vi "PIV_transform.vi"(8 "error in (no error)":errorcluster, 11 "raw":T1) -> (0 "error out":errorcluster={"status"=TRUE, "code"=1671, "source"="Python Node in PIV_Pixel.vi->LabVIEW_GUI.vi<APPEND>\n\nModule Path: /Users/crogers/Desktop/PIV/LabVIEW/subs/code.py\nFunction Name: piv\nPython returned the following error: <class 'OSError'>\nImageIO does not generally support reading folders. Limited support may be available via specific plugins. Specify the plugin explicitly using the `plugin` kwarg, e.g. `plugin='DICOM'`\n\n\n Call Stack information:\n['Traceback (most recent call last):\n', '  File \"/Users/crogers/Desktop/PIV/LabVIEW/subs/code.py\", line 8, in piv\n    frame_a = tools.imread(path_t)\n', '  File \"/Users/crogers/Library/Python/3.10/lib/python/site-packages/openpiv/tools.py\", line 337, in imread\n    im = _imread(filename)\n', '  File \"/Users/crogers/Library/Python/3.10/lib/python/site-packages/imageio/v3.py\", line 53, in imread\n    with imopen(uri, \"r\", **plugin_kwargs) as img_file:\n', '  File \"/Users/crogers/Library/Python/3.10/lib/python/site-packages/imageio/core/imopen.py\", line 223, in imopen\n    raise err_type(err_msg)\n', \"OSError: ImageIO does not generally support reading folders. Limited support may be available via specific plugins. Specify the plugin explicitly using the `plugin` kwarg, e.g. `plugin='DICOM'`\n\"]"}, 3 "interpolated":T1)   [LabVIEW 2025]
uses:
  PIV_velocities.ctl
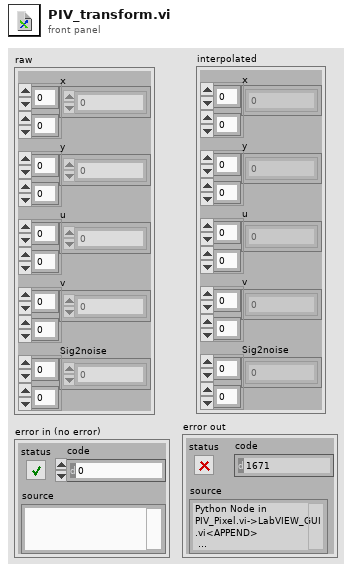
[diagram p1: front panel]
types:
  T1 = typedef "PIV_velocities.ctl" = cluster{"x":dbl[][], "y":dbl[][], "u":dbl[][], "v":dbl[][], "Sig2noise":dbl[][]}
  T2 = cluster{"x":dbl[][], "y":dbl[][], "u3":dbl[][], "v3":dbl[][]}
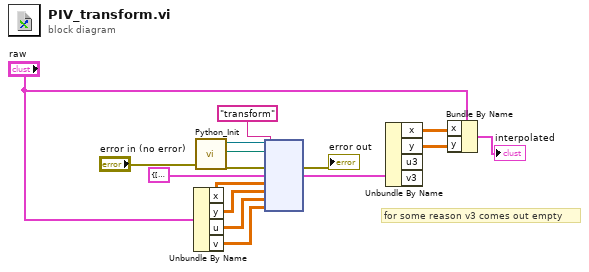
[diagram p0: block diagram]
diagram:
  # "for some reason v3 comes out empty"
  n1 = Unbundle By Name("raw") -> ("x"=w6:dbl[][], "y"=w5:dbl[][], "u"=w4:dbl[][], "v"=w3:dbl[][])
  n2 = call "Python_Init.vi"("error in (no error)"="error in (no error)") -> ("Refnum out"=w15:refnum<k35>, "code"=w12:path, "error out"=w16:errorcluster)  [unwired: 3 in]
  n3 = node(w15, w12, "transform" ("function name"), w16, T2 {"x"=[], "y"=[], "u3"=[], "v3"=[]}, w6, w5, w4, w3) -> (→"error out":errorcluster, w7:T2)  [unwired: 4 in, 3 out]
  n4 = Unbundle By Name(w7) -> ("x"=w2:dbl[][], "y"=w1:dbl[][])  [unwired: 2 out]
  n5 = Bundle By Name(cluster="raw", "x"=w2, "y"=w1) -> (→"interpolated":T1)
